vi "Esercitazione 1 - Somma, diff, prod, div.vi"() -> ()   [LabVIEW 2018]
panel:
  in  "Operatore 3":i32
  out "Compound":dbl
  out "Media":dbl
  out "Divisione":dbl
  out "Prodotto":i32
  out "Differenza":i32
  out "Somma":i32
  in  "Operatore 2":i32
  in  "Operatore 1":i32
  # "somma, diff, divisione, prodotto, compound"
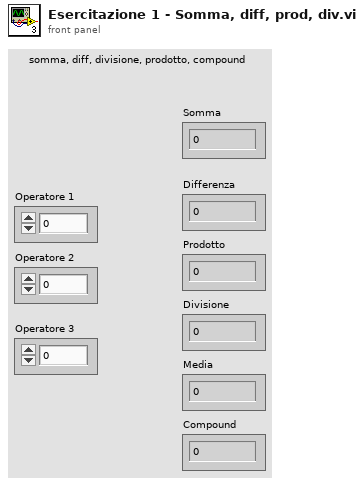
[diagram p1: front panel]
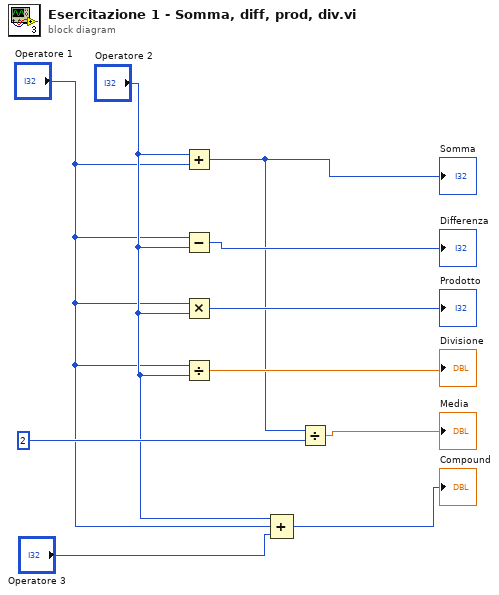
[diagram p0: block diagram]
diagram:
  n1 = Add(x="Operatore 2", y="Operatore 1") -> (x+y=w6:i32)
  "Somma" <- w6
  n2 = Subtract(x="Operatore 1", y="Operatore 2") -> (x-y=→"Differenza":i32)
  n3 = Multiply(x="Operatore 1", y="Operatore 2") -> (x*y=→"Prodotto":i32)
  n4 = Divide(x="Operatore 1", y="Operatore 2") -> (x/y=→"Divisione":dbl)
  n5 = Compound Arithmetic op=ADD("Operatore 2", "Operatore 1", "Operatore 3") -> (→"Compound":i32)
  n6 = Divide(x=w6, y=2) -> (x/y=→"Media":dbl)
